vi "lvUpdateProjectFiles.vi"() -> ()   [LabVIEW 2015, in "veristand-steps-codegen.lvlib"]
uses:
  veristand-steps-codegen.lvlib
  <vilib>/Wiresmith Technology/LabVIEW CLI/CLI Class/CLI.lvclass
panel:
  out "error out":errorcluster
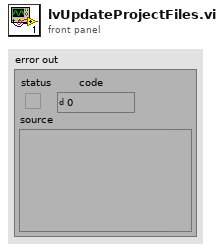
[diagram p1: front panel]
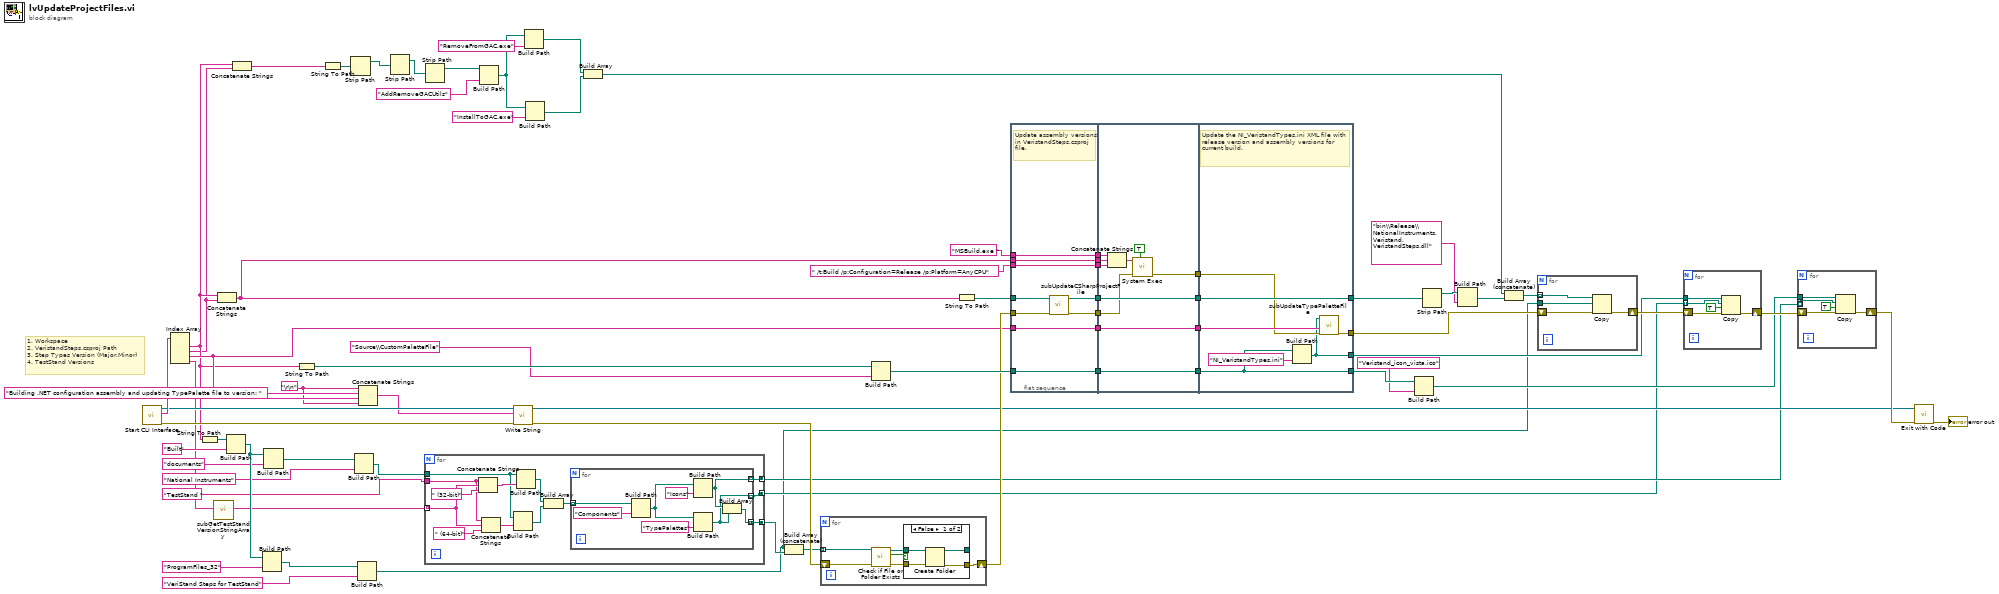
[diagram p0: block diagram]
diagram:
  w44 = "\r\n"
  # "1. Workspace\n2. VeristandSteps.csproj Path\n3. Step Types Version (Major.Minor)\n4. TestStand Versions"
  n1 = call <vilib>:"Start CLI Interface.vi"() -> ("error out"=w51:errorcluster, "Custom Parameters"=w73:string[], "CLI out"=w50:refnum<class "CLI.lvclass">)  [unwired: 9 in]
  n2 = Index Array(array=w73) -> (element #1=w11:string, element #2=w10:string, element #3=w47:string, element #4=w36:string)  [unwired: 4 in]
  n3 = String To Path(string=w11) -> (path=w71:path)
  n4 = call "subGetTestStandVersionStringArray.vi"("TestStand Version String"=w36) -> ("TestStand Version String Array"=w35:string[])  [unwired: 10 in]
  n5 = Concatenate Strings(w11, w10) -> (w64:string)
  n6 = Build Path(base path=w71, name or relative path="Built") -> (appended path=w40:path)
  n7 = Concatenate Strings(w11, w10) -> (w9:string)
  n8 = Build Path(base path=w40, name or relative path="ProgramFiles_32") -> (appended path=w33:path)
  n9 = Build Path(base path=w40, name or relative path="documents") -> (appended path=w38:path)
  n10 = String To Path(string=w11) -> (path=w67:path)
  n11 = String To Path(string=w9) -> (path=w24:path)
  n12 = Strip Path(path=w24) -> (stripped path=w23:path)  [unwired: 1 out]
  n13 = Build Path(base path=w38, name or relative path="National Instruments") -> (appended path=w29:path)
  n14 = Build Path(base path=w33, name or relative path="VeriStand Steps for TestStand") -> (appended path=w1:path)
  n15 = Concatenate Strings(w44, "Building .NET configuration assembly and updating TypePalette file to version: " ("string"), w47, w44) -> (w46:string)
  n16 = Strip Path(path=w23) -> (stripped path=w13:path)  [unwired: 1 out]
  n17 = for {
    tunnel: w35 -> [w85] mode=indexing
    tunnel: w29 -> [w82]
    tunnel: "TestStand " ("name or relative path") -> [w81]
    tunnel: [w77] -> w8 mode=concatenating
    tunnel: [w76] -> w3 mode=concatenating
    tunnel: [w75] -> w2 mode=concatenating
    n18 = Concatenate Strings(w81, w85, " (32-bit)" ("string")) -> (w83:string)
    n19 = Concatenate Strings(w81, w85, " (64-bit)" ("string")) -> (w84:string)
    n20 = Build Path(base path=w82, name or relative path=w84) -> (appended path=w79:path)
    n21 = Build Path(base path=w82, name or relative path=w83) -> (appended path=w80:path)
    n22 = Build Array(w80, w79) -> (w78:path[])
    n23 = for {
      tunnel: w78 -> [w95] mode=indexing
      tunnel: [w90] -> w77 mode=concatenating
      tunnel: [w89] -> w76 mode=indexing
      tunnel: [w88] -> w75 mode=indexing
      n24 = Build Path(base path=w95, name or relative path="Components") -> (appended path=w92:path)
      n25 = Build Path(base path=w92, name or relative path="Icons") -> (appended path=w89:path)
      n26 = Build Path(base path=w92, name or relative path="TypePalettes") -> (appended path=w88:path)
      n27 = Build Array(w89, w88) -> (w90:path[])
    }
  }
  n28 = Strip Path(path=w13) -> (stripped path=w12:path)  [unwired: 1 out]
  n29 = Build Path(base path=w12, name or relative path="AddRemoveGACUtils") -> (appended path=w20:path)
  n30 = call <vilib>:"Write String.vi"("error in (no error)"=w51, "Text to Write"=w46, "CLI in"=w50) -> ("error out"=w49:errorcluster, "CLI out"=w48:refnum<class "CLI.lvclass">)  [unwired: 7 in]
  n31 = Build Path(base path=w20, name or relative path="RemoveFromGAC.exe") -> (appended path=w17:path)
  n32 = Build Path(base path=w20, name or relative path="InstallToGAC.exe") -> (appended path=w16:path)
  n33 = Build Array(w17, w16) -> (w15:path[])
  n34 = Build Array (concatenate)(w1, w8) -> (w31:path[])
  n35 = for {
    shift-right: [w98] -> w54
    shift-left: w49 -> [w97]
    tunnel: w31 -> [w96] mode=indexing
    n36 = call <vilib>:"Check if File or Folder Exists.vi"("error in (no error)"=w97, "path"=w96) -> ("error out"=w101:errorcluster, "file or folder exists?"=w99:bool, "dup path"=w100:path)  [unwired: 7 in]
    n37 = case shown="False" w99 {
      tunnel: w101 -> [w105 w106]
      tunnel: w100 -> [w104 w107]
      tunnel: [w103 w106] -> w98
      tunnel: [w102 w107] -> _
      frame False {
        n38 = Create Folder(path (use dialog)=w104, error in=w105) -> (created path=w102:path, error out=w103:errorcluster)  [unwired: 1 in, 1 out]
      }
      frame True {
      }
    }
  }
  n39 = Build Path(base path=w67, name or relative path="Source\\CustomPaletteFile") -> (appended path=w56:path)
  n40 = String To Path(string=w64) -> (path=w60:path)
  n41 = flat-sequence {
    tunnel: w64 -> [w114]
    tunnel: " /t:Build /p:Configuration=Release /p:Platform=AnyCPU" ("string") -> [w115]
    tunnel: "MSBuild.exe " -> [w116]
    tunnel: [w116] -> w63
    tunnel: [w115] -> w62
    tunnel: [w114] -> w61
    tunnel: w60 -> [w113]
    tunnel: [w112] -> w59
    tunnel: [w111] -> w58
    tunnel: w56 -> [w110]
    tunnel: [w110] -> w55
    tunnel: w54 -> [w109]
    tunnel: w47 -> [w108]
    tunnel: [w108] -> w53
    tunnel: [w126] -> w43
    tunnel: [w125] -> w42
    tunnel: [w124] -> w41
    tunnel: w53 -> [w124]
    tunnel: w55 -> [w125]
    tunnel: w58 -> [w126]
    tunnel: w59 -> [w118]
    tunnel: w61 -> [w120]
    tunnel: w62 -> [w121]
    tunnel: w63 -> [w122]
    tunnel: [w117] -> w30
    tunnel: [w133] -> w57
    tunnel: w43 -> [w133]
    tunnel: w42 -> [w130]
    tunnel: [w132] -> w25
    tunnel: [w130] -> w27
    tunnel: w41 -> [w129]
    tunnel: w30 -> [w128]
    tunnel: [w127] -> w5
    frame #0 {
      # "Update assembly versions in VeristandSteps.csproj file."
      n42 = call "subUpdateCSharpProjectFile.vi"("error in (no error)"=w109, ".csproj path"=w113) -> ("error out"=w112:errorcluster, ".csproj path out"=w111:path)  [unwired: 8 in]
    }
    frame #1 {
      n43 = Concatenate Strings(w122, w120, w121) -> (w119:string)
      n44 = call <vilib>:"System Exec.vi"("wait until completion? (T)"=TRUE, "error in (no error)"=w118, "command line"=w119) -> ("error out"=w117:errorcluster)  [unwired: 5 in, 3 out]
    }
    frame #2 {
      # "Update the NI_VeristandTypes.ini XML file with release version and assembly versions for current build."
      n45 = Build Path(base path=w130, name or relative path="NI_VeristandTypes.ini") -> (appended path=w127:path)
      n46 = call "subUpdateTypePaletteFile.vi"("error in (no error)"=w128, "Step Types Version"=w129, "TypePalette .ini file location"=w127) -> ("error out"=w132:errorcluster)  [unwired: 8 in]
    }
  }
  n47 = Build Path(base path=w27, name or relative path="Veristand_icon_vista.ico") -> (appended path=w4:path)
  n48 = Strip Path(path=w57) -> (stripped path=w69:path)  [unwired: 1 out]
  n49 = Build Path(base path=w69, name or relative path="bin\\Release\\NationalInstruments.Veristand.VeristandSteps.dll") -> (appended path=w21:path)
  n50 = Build Array (concatenate)(w15, w21) -> (w14:path[])
  n51 = for {
    shift-right: [w137] -> w7
    shift-left: w25 -> [w136]
    tunnel: w14 -> [w135] mode=indexing
    tunnel: w1 -> [w134]
    n52 = Copy(8:w136, 10:w134, 11:w135) -> (0:w137:errorcluster)  [unwired: 2 in, 2 out]
  }
  n53 = for {
    shift-right: [w142] -> w6
    shift-left: w7 -> [w141]
    tunnel: w5 -> [w139]
    tunnel: w2 -> [w138] mode=indexing
    n54 = Copy(8:w141, 9:TRUE ("overwrite (F)"), 10:w138, 11:w139) -> (0:w142:errorcluster)  [unwired: 1 in, 2 out]
  }
  n55 = for {
    shift-right: [w147] -> w65
    shift-left: w6 -> [w146]
    tunnel: w4 -> [w144]
    tunnel: w3 -> [w143] mode=indexing
    n56 = Copy(8:w146, 9:TRUE ("overwrite (F)"), 10:w143, 11:w144) -> (0:w147:errorcluster)  [unwired: 1 in, 2 out]
  }
  n57 = call <vilib>:"Exit with Code.vi"("error in (no error)"=w65, "CLI in"=w48) -> ("error out"=→"error out":errorcluster)  [unwired: 9 in]
